vi "Process Primary.vi"(11 "Chmmr in":refnum<class "Chmmr.lvclass">) -> (2 "Laser":refnum<class "Element.lvclass">[](array[class]), 3 "Chmmr out":refnum<class "Chmmr.lvclass">)   [LabVIEW 2021, in "Chmmr.lvclass"]
uses:
  Chmmr.lvclass
  Element/Element.lvclass
  Chmmr.lvclass/Chmmr.ctl
  Weapons/Laser/Laser.lvclass
  Motion/Motion.lvclass
  Re-use Libraries/Vector 2D/Vector 2D.lvclass
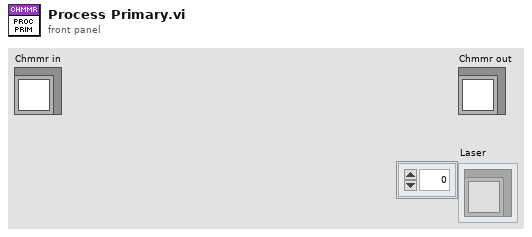
[diagram p1: front panel]
types:
  T1 = typedef "Element.lvclass/Player Type.ctl" = enum16{"Neutral", "Player 1", "Player 2"}
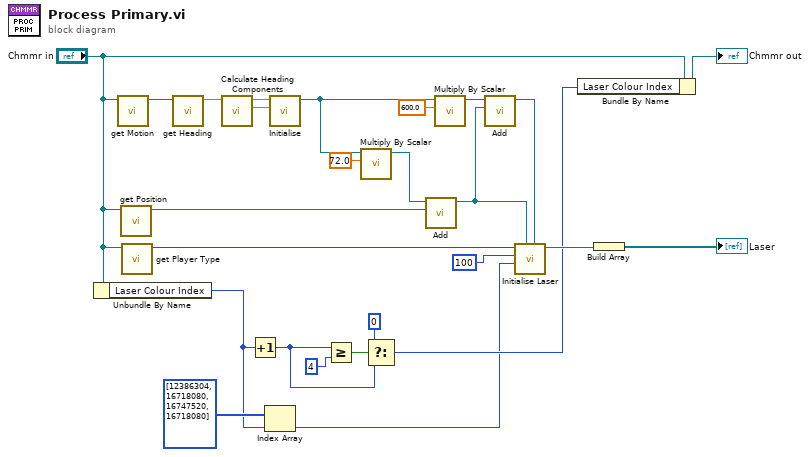
[diagram p0: block diagram]
diagram:
  n1 = Unbundle By Name("Chmmr in") -> ("Laser Colour Index"=w9:i32)
  n2 = call "get Motion.vi"("Element in"="Chmmr in") -> ("Motion"=w24:refnum<class "Motion.lvclass">)  [unwired: 10 in]
  n3 = call "get Position.vi"("Element in"="Chmmr in") -> ("Position"=w14:refnum<class "Vector 2D.lvclass">)  [unwired: 10 in]
  n4 = call "get Player Type.vi"("Element in"="Chmmr in") -> ("Player Type"=w1:T1)  [unwired: 10 in]
  n5 = call "get Heading.vi"("Motion in"=w24) -> ("Heading [deg]"=w23:sgl)  [unwired: 10 in]
  n6 = call "Calculate Heading Components.vi"("Heading In [deg]"=w23) -> ("Sin Heading"=w21:sgl, "Cos Heading"=w22:sgl)  [unwired: 9 in]
  n7 = Increment(x=w9) -> (x+1=w6:i32)
  n8 = Index Array(array=u32[] [12386304, 16718080, 16747520, 16718080], index=w9) -> (element=w3:u32)
  n9 = call "Initialise.vi"("y"=w21, "x"=w22) -> ("Vector 2D out"=w15:refnum<class "Vector 2D.lvclass">)  [unwired: 9 in]
  n10 = Greater Or Equal?(x=w6, y=4) -> (x >= y?=w7:bool)
  n11 = call "Multiply By Scalar.vi"("x"=sgl 72.0, "A"=w15) -> ("Ax"=w13:refnum<class "Vector 2D.lvclass">)  [unwired: 9 in]
  n12 = Select(t=0 ("y"), s=w7, f=w6) -> (s? t:f=w4:i32)
  n13 = call "Add.vi"("B"=w14, "A"=w13) -> ("A+B"=w12:refnum<class "Vector 2D.lvclass">)  [unwired: 9 in]
  n14 = call "Multiply By Scalar.vi"("x"=sgl 600.0, "A"=w15) -> ("Ax"=w18:refnum<class "Vector 2D.lvclass">)  [unwired: 9 in]
  n15 = call "Add.vi"("B"=w12, "A"=w18) -> ("A+B"=w17:refnum<class "Vector 2D.lvclass">)  [unwired: 9 in]
  n16 = call "Initialise Laser.vi"("Endpoint"=w17, "Origin"=w12, "Colour"=w3, "Damage"=100, "Player Type"=w1) -> ("Laser out"=w26:refnum<class "Laser.lvclass">)  [unwired: 6 in]
  n17 = Bundle By Name(cluster="Chmmr in", "Laser Colour Index"=w4) -> (→"Chmmr out":refnum<class "Chmmr.lvclass">)
  n18 = Build Array(w26) -> (→"Laser":refnum<class "Laser.lvclass">[])
